vi "Fibre Flow Laser_Control.vi"() -> ()   [LabVIEW 2020]
uses:
  ADAM Client/Sub VIs/ADAM Controls/Update_scan_value.ctl
  Anemometry/Anemometry Sub Vis/File/Setup_Filetype.ctl
  Anemometry/Anemometry Sub Vis/Globals/LDA_global.vi
panel:
  out "BSA IP and Channels":string[](array[string])
  out "Setup String":string
  out "Setup Filename":string
  in  "Update BSA Settings":bool
  out "reference out":refnum<k7>
  in  "SysMon":refnum<k7>(container)
  in  "Stop BSA Monitor":bool
  in  "Start BSA Monitor":bool
  out "Laser Control Error":errorcluster
  out "BSA Error":errorcluster
  in  "Freqency Shift Enable?":bool
  in  "Control Laser":bool
  in  "Mode":T1(ring)
  in  "Set Power (mW)":dbl
  in  "Laser":i32(listbox)
  in  "Seconds before Update":u32=30
  out "Numeric":i32
  in  "stop":bool
  out "Status":string[][](array[string])
  out "Laser Status error":errorcluster
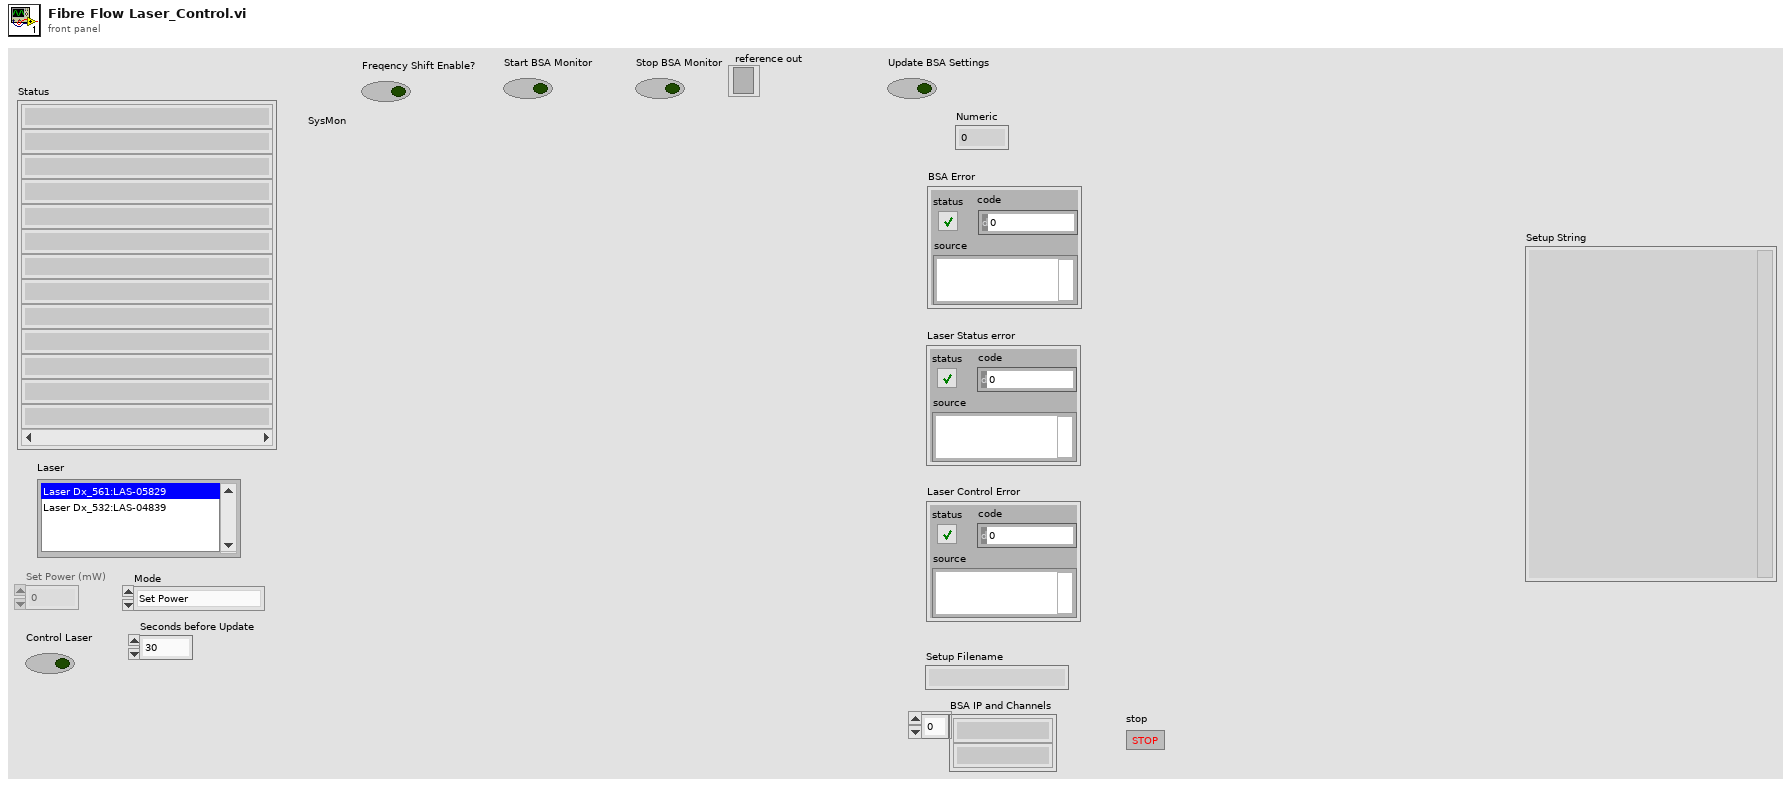
[diagram p1: front panel]
types:
  T1 = enum16{"Set Power", "Turn Laser On", "Turn Laser Off", "Shutter Open", "Shutter Closed", "Attenuated"}
  T2 = typedef "Update_scan_value.ctl" = cluster{"Channel Name":string, "New Value":dbl}
  T3 = enum16{"Zero or one", "One", "Zero or more", "One or more"}
  T4 = typedef "Setup_Filetype.ctl" = enum16{"Measurement Setups", "Calibration Setups", "General", "Results File Plotter Setups", "Speed Calib Tweaks"}
  T5 = enum8{"Enabled", "Disabled", "Disabled and Grayed Out"}
  T6 = typedef "LDA_Channel.ctl" = cluster{"Wavelength (nm)":dbl, "Vel Comp":string, "Max Velocity":dbl, "Min Velocity":dbl, "Max Record length":u16, "Signal gain (dB)":i16, "High voltage":i16, "Optics Conversion Factor":dbl, "Min Record length":u16, "Multiply Velocity by -1":bool, "Signal to Noise Ratio":string, "Validation Ratio":string, "Probe":string, "Laser":string, "BSA":string, "Lense":string, "Beam Separation (mm)":dbl, "Focal Length (mm)":dbl, "COLOUR":u32, "BSA IP":string, "Velocity Range (m/s)":dbl, "Centre Velocity (m/s)":dbl, "Unshifted mW":dbl, "Shifted mW":dbl, "Bandwidth Hz":dbl, "Req Sampling Rate Hz":dbl, "Ch":i32, "CenterFreq Hz":dbl, "Laser IP":string}
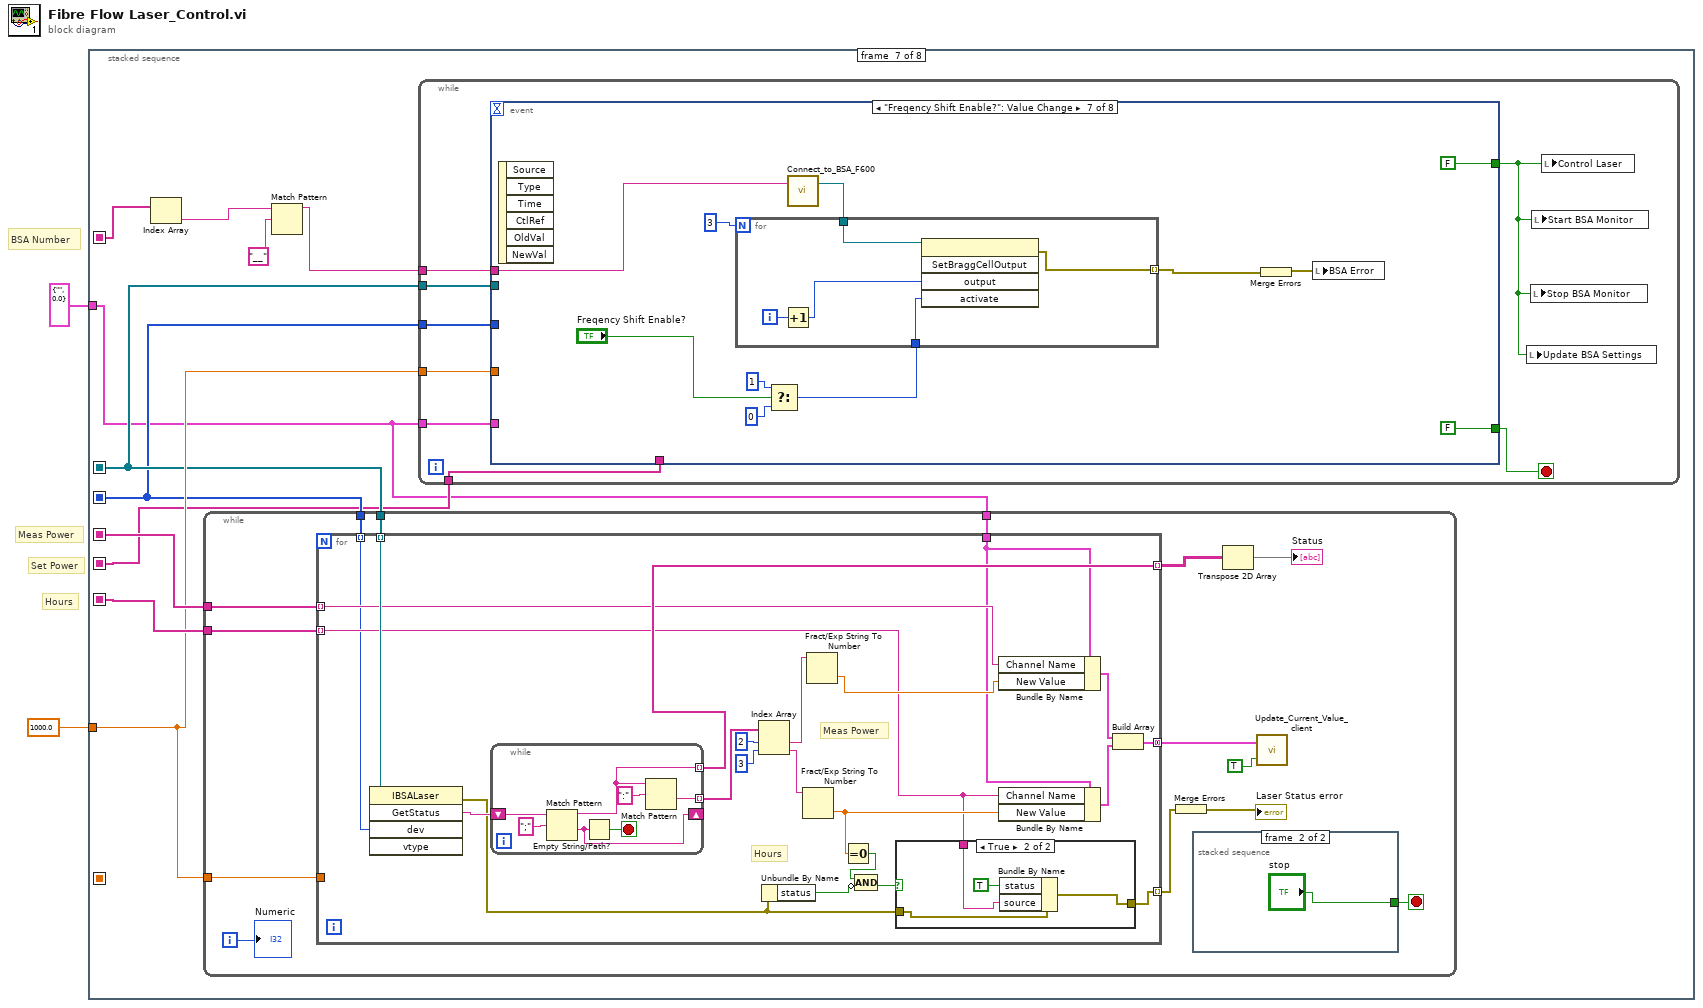
[diagram p0: block diagram]
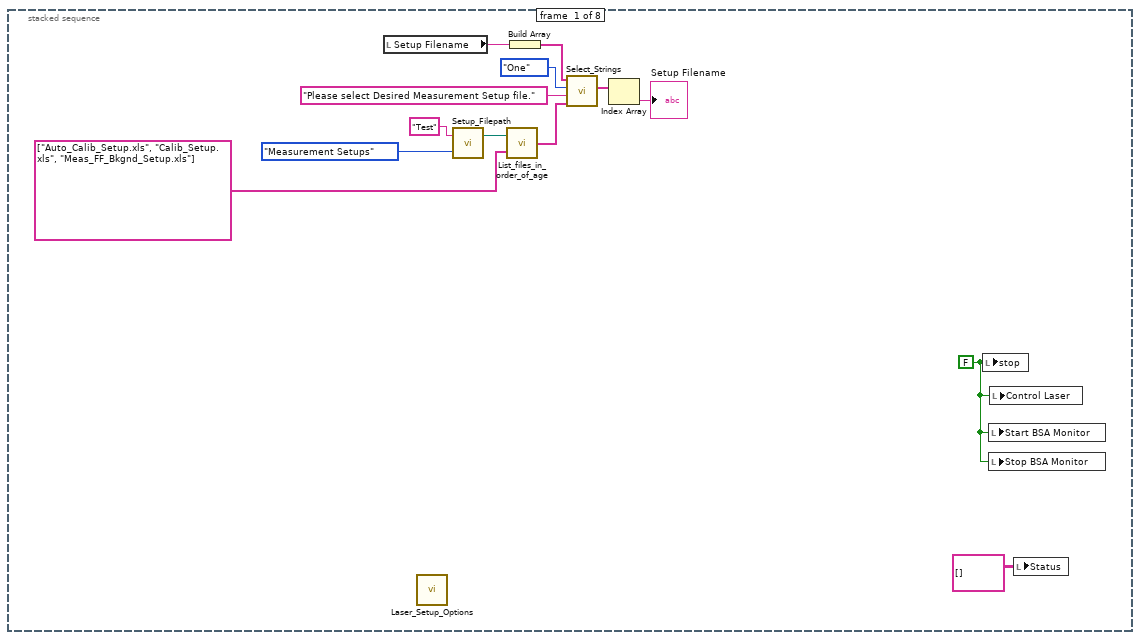
[diagram p2: hidden frame]
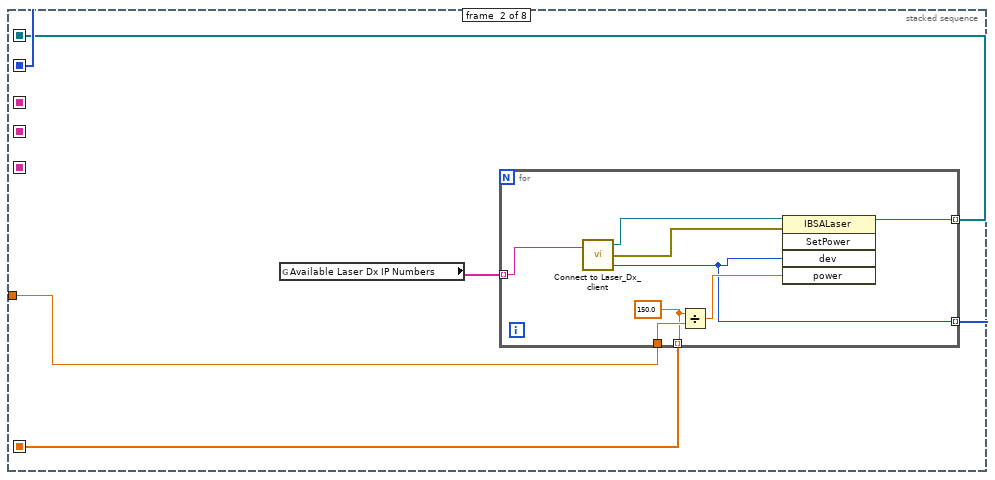
[diagram p3: hidden frame]
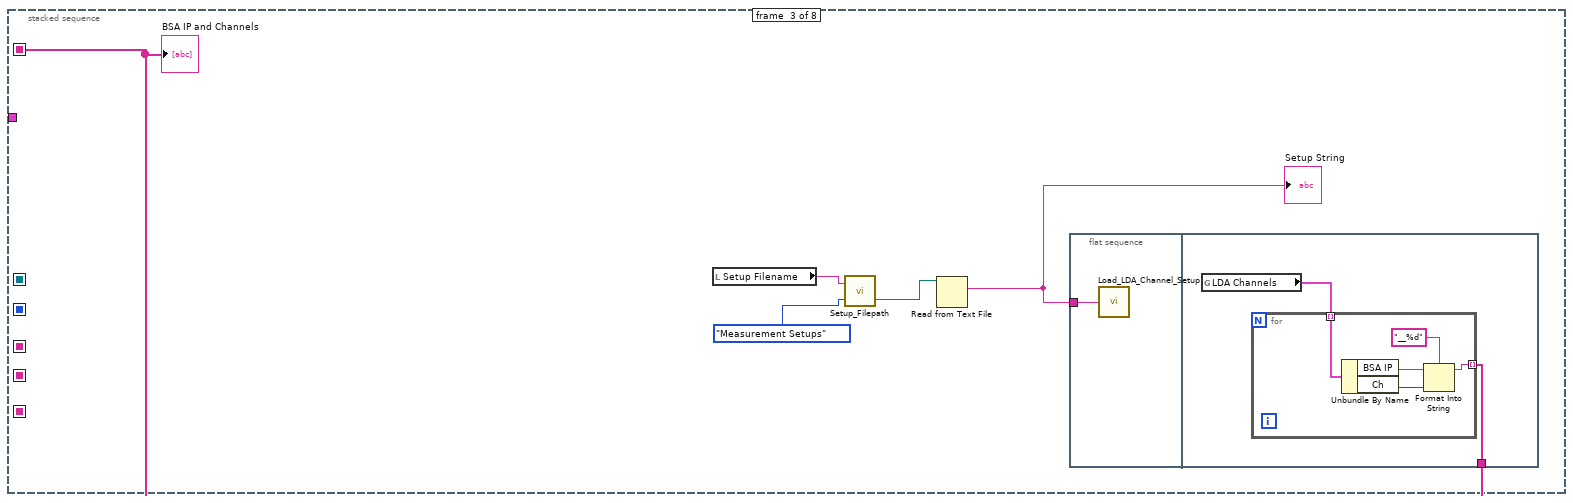
[diagram p4: hidden frame]
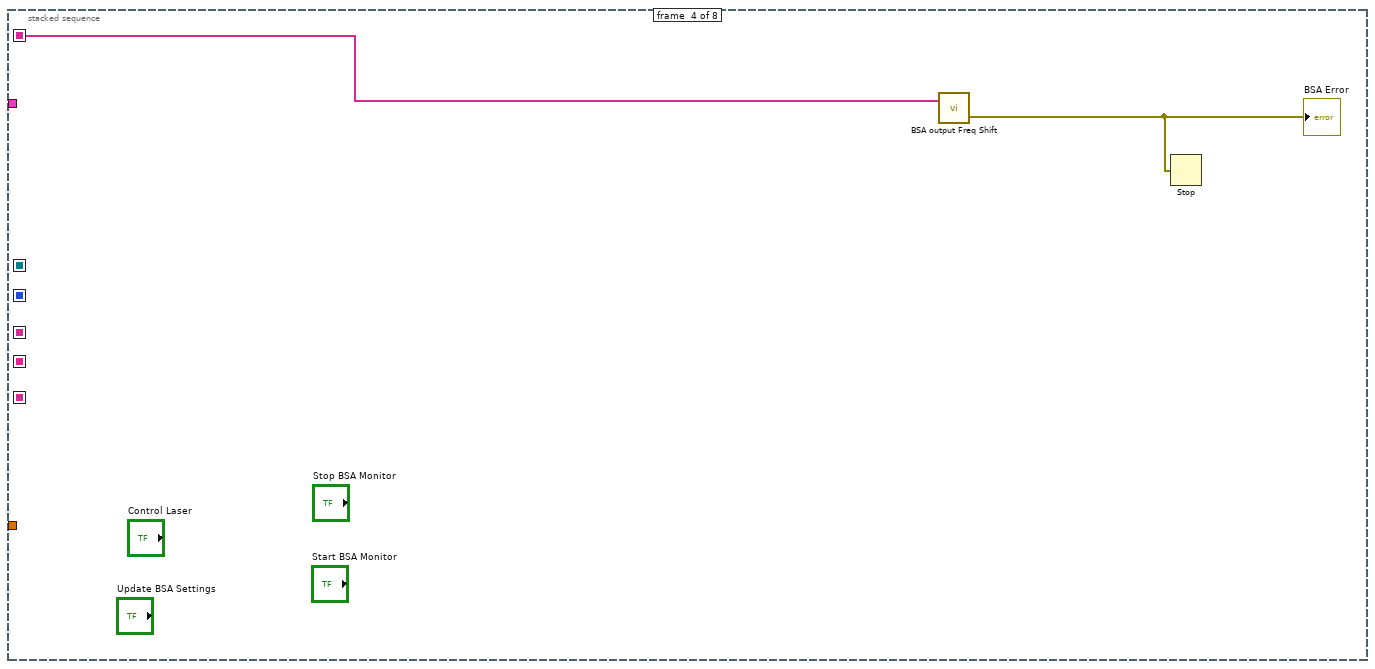
[diagram p5: hidden frame]
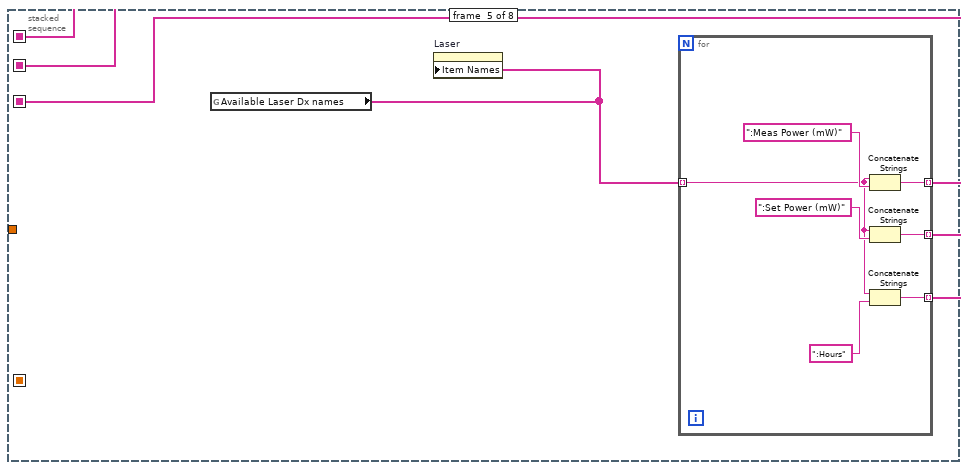
[diagram p6: hidden frame]
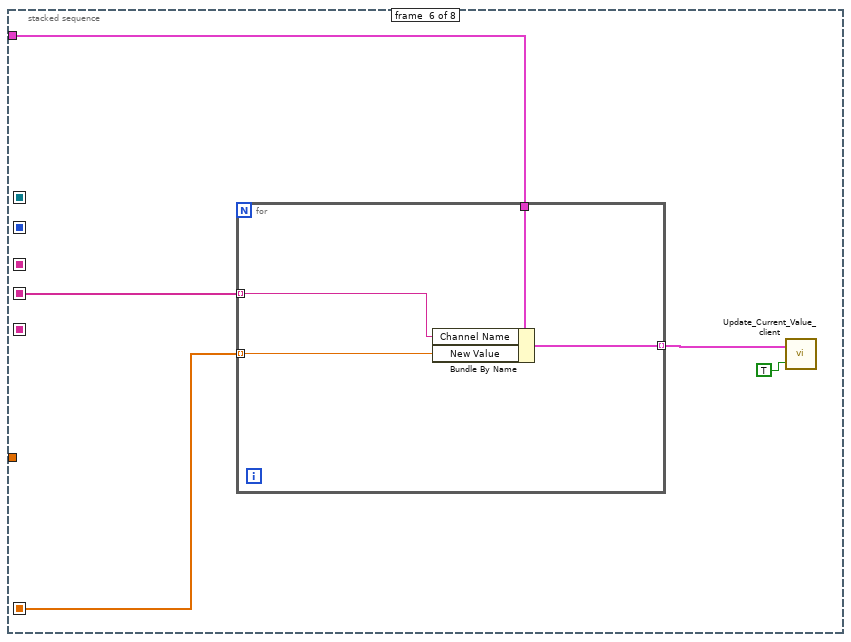
[diagram p7: hidden frame]
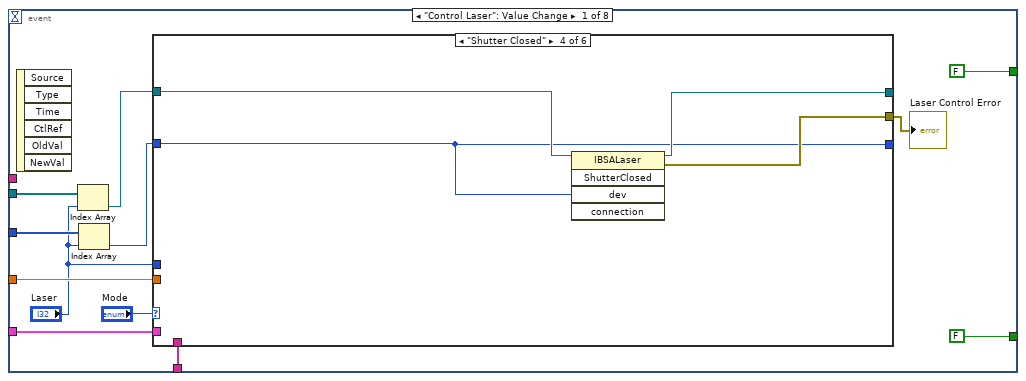
[diagram p8: hidden frame]
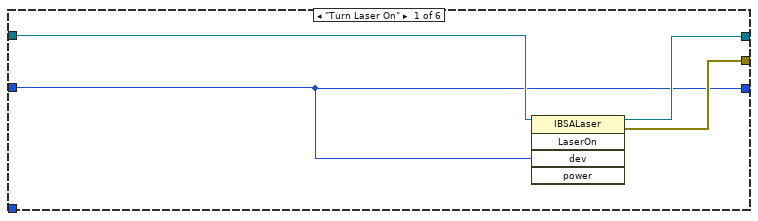
[diagram p9: hidden frame]
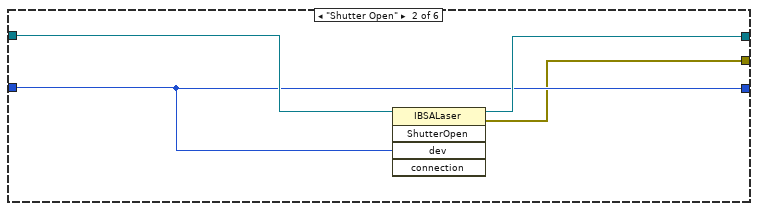
[diagram p10: hidden frame]
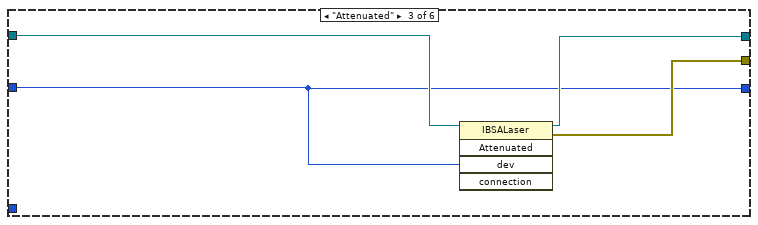
[diagram p11: hidden frame]
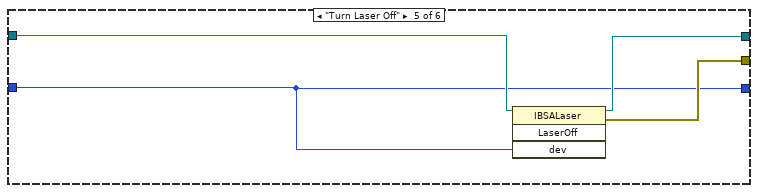
[diagram p12: hidden frame]
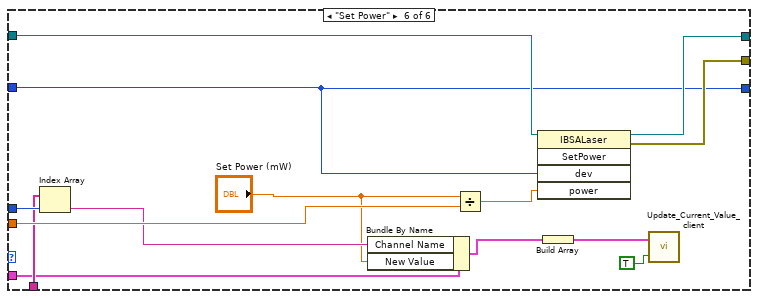
[diagram p13: hidden frame]
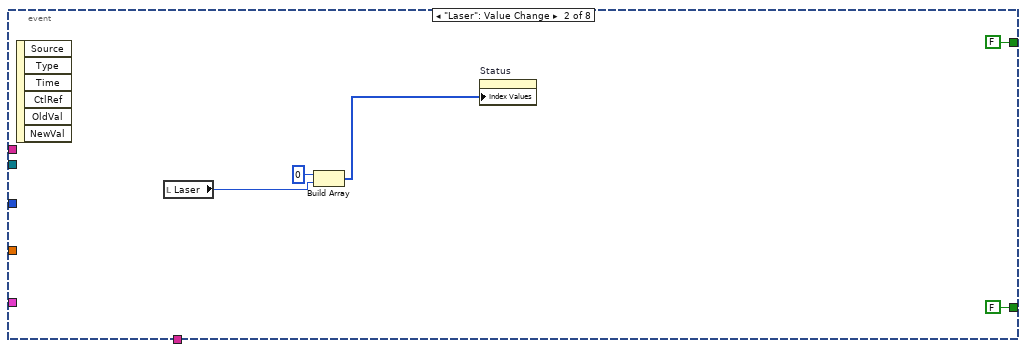
[diagram p14: hidden frame]
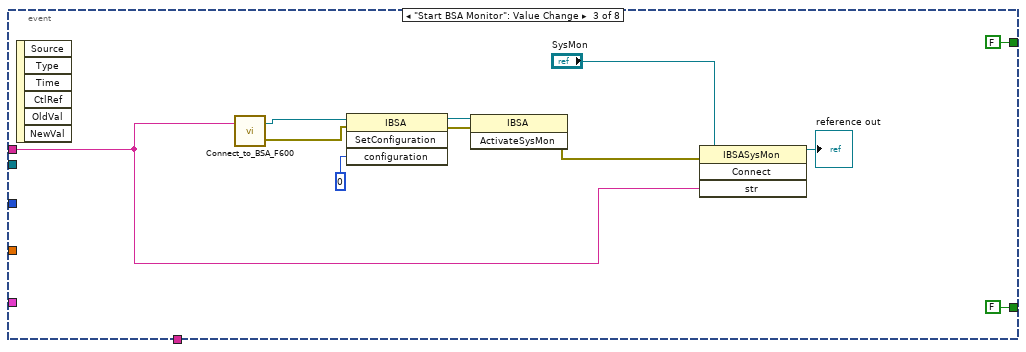
[diagram p15: hidden frame]
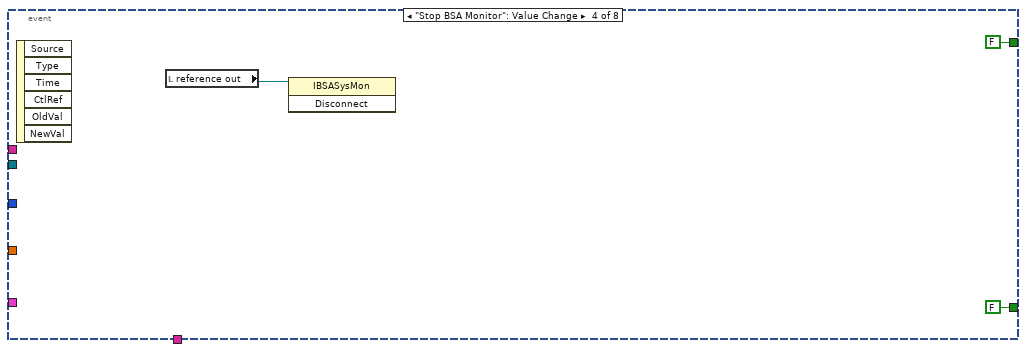
[diagram p16: hidden frame]
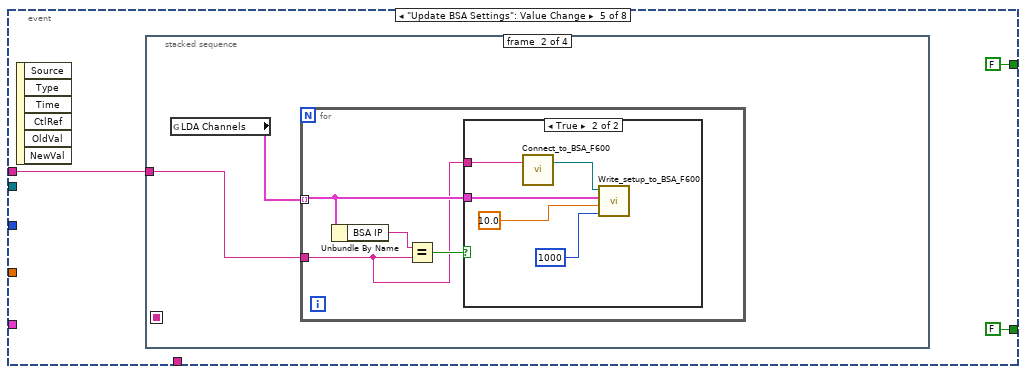
[diagram p17: hidden frame]
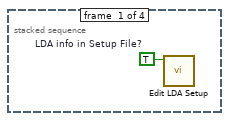
[diagram p18: hidden frame]
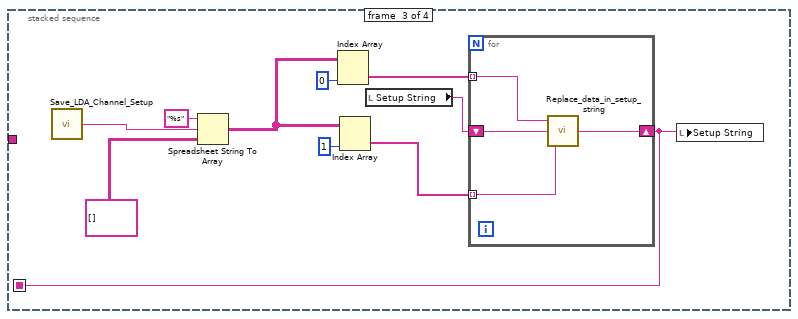
[diagram p20: hidden frame]
diagram:
  # "BSA Number"
  # "Hours"
  # "Set Power"
  # "Meas Power"
  n1 = stacked-sequence {
    seq-local: [_ w16 _ _ _ _ _ _] -> [_ _ _ _ _ _ w71 _]
    seq-local: [_ w20 _ _ _ _ _ _] -> [_ _ _ _ _ _ w70 _]
    seq-local: [_ _ _ _ w47 _ _ _] -> [_ _ _ _ _ _ w74 w268]
    seq-local: [_ _ _ _ w46 _ _ _] -> [_ _ _ _ _ w58 w69 w267]
    seq-local: [_ _ _ _ w45 _ _ _] -> [_ _ _ _ _ _ w73 w266]
    seq-local: [_ w18 _ _ _ _ _ _] -> [_ _ _ _ _ w57 _ _]
    seq-local: [_ _ w30 _ _ _ _ _] -> [_ _ _ w42 _ _ w65 _]
    tunnel: 1000.0 ("y") -> [_ w19 _ _ _ _ w72 _]
    tunnel: T2 {"Channel Name"="", "New Value"=0.0} ("Update Scan Value Cluster") -> [_ _ _ _ _ w55 w68 w264]
    frame #0 {
      w3 = FALSE ("stop")
      n2 = local read "Setup Filename"() -> (w12:string)
      n3 = call "Laser_Setup_Options.vi"() -> ()  [unwired: 5 in, 4 out]
      n4 = call "Setup_Filepath.vi"("Setup File Type"=Setup_Filetype."Measurement Setups", "Filename in"="Test") -> ("Directory"=w15:path)  [unwired: 1 out]
      n5 = call "List_files_in_order_of_age.vi"("Files to Hide"=string[] ["Auto_Calib_Setup.xls", "Calib_Setup.xls", "Meas_FF_Bkgnd_Setup.xls"] ("file names"), "Folder"=w15) -> ("file names"=w14:string[])
      n6 = Build Array(w12) -> (w11:string[])
      n7 = call "Select_Strings.vi"("Available Ch names"=w14, "Message"="Please select Desired Measurement Setup file.", "Selector mode"=T3."One", "Desired Ch names (in)"=w11) -> ("Selected Channel Names"=w13:string[])  [unwired: 2 in, 2 out]
      n8 = Index Array(array=w13) -> (element=→"Setup Filename":string)  [unwired: 1 in]
      n9 = local write "stop"(w3) -> ()
      n10 = local write "Start BSA Monitor"(w3) -> ()
      n11 = local write "Stop BSA Monitor"(w3) -> ()
      n12 = local write "Control Laser"(w3) -> ()
      n13 = local write "Status"(string[][] [] ("Status")) -> ()
    }
    frame #1 {
      n14 = global read "LDA_global.vi" "Available Laser Dx IP Numbers"() -> (w17:string[])
      n15 = for {
        tunnel: w17 -> [w24] mode=indexing
        tunnel: [w28] -> w16 mode=indexing
        tunnel: [w21] -> w20 mode=indexing
        tunnel: w19 -> [w27]
        tunnel: [w25] -> w18 mode=indexing
        w25 = 150.0 ("power")
        n16 = call "Connect to Laser_Dx_client.vi"("Laser IP Number"=w24) -> ("Laser_Dx"=w23:refnum<k7>, "error out"=w22:errorcluster, "Channel"=w21:i64)  [unwired: 1 in]
        n17 = Divide(x=w25, y=w27) -> (x/y=w26:dbl)
        n18 = invoke class="IBSALaser" method="SetPower"(reference=w23, error in=w22, "dev"=w21, "power"=w26) -> (reference out=w28:refnum<k7>)  [unwired: 1 in, 4 out]
      }
    }
    frame #2 {
      n19 = local read "Setup Filename"() -> (w29:string)
      n20 = call "Setup_Filepath.vi"("Setup File Type"=Setup_Filetype."Measurement Setups", "Filename in"=w29) -> ("Filename Out"=w32:path)  [unwired: 1 out]
      n21 = Read from Text File(file (use dialog)=w32) -> (text=w31:string)  [unwired: 3 in, 3 out]
      "Setup String" <- w31
      n22 = flat-sequence {
        tunnel: w31 -> [w34]
        tunnel: [w36] -> w30
        frame #0 {
          n23 = call "Load_LDA_Channel_Setup.vi"("Setup file string"=w34) -> ()  [unwired: 1 in]
        }
        frame #1 {
          n24 = global read "LDA_global.vi" "LDA Channels"() -> (w35:T6[])
          n25 = for {
            tunnel: [w37] -> w36 mode=indexing
            tunnel: w35 -> [w41] mode=indexing
            n26 = Unbundle By Name(w41) -> ("BSA IP"=w39:string, "Ch"=w40:i32)
            n27 = Format Into String(format string="__%d", initial string=w39, w40) -> (resulting string=w37:string)  [unwired: 1 in, 1 out]
          }
        }
      }
      "BSA IP and Channels" <- w30
    }
    frame #3 {
      n28 = call "BSA output Freq Shift.vi"("BSAIP__ChNum"=w42) -> ("BSA Error"=w43:errorcluster)  [unwired: 2 in]
      "BSA Error" <- w43
      n29 = Stop(stop? (T)=w43) -> ()
    }
    frame #4 {
      n30 = global read "LDA_global.vi" "Available Laser Dx names"() -> (w44:string[])
      n31 = property on="Laser" class="LstBox (strict)"("Item Names"=w44) -> ()  [unwired: 2 in, 2 out]
      n32 = for {
        tunnel: [w51] -> w47 mode=indexing
        tunnel: [w50] -> w46 mode=indexing
        tunnel: [w49] -> w45 mode=indexing
        tunnel: w44 -> [w48] mode=indexing
        n33 = Concatenate Strings(w48, ":Meas Power (mW)" ("string")) -> (w51:string)
        n34 = Concatenate Strings(w48, ":Set Power (mW)" ("string")) -> (w50:string)
        n35 = Concatenate Strings(w48, ":Hours" ("string")) -> (w49:string)
      }
    }
    frame #5 {
      n36 = for {
        tunnel: w58 -> [w63] mode=indexing
        tunnel: w57 -> [w62] mode=indexing
        tunnel: [w61] -> w56 mode=indexing
        tunnel: w55 -> [w60]
        n37 = Bundle By Name(cluster=w60, "Channel Name"=w63, "New Value"=w62) -> (w61:T2)
      }
      n38 = call "Update_Current_Value_client.vi"("Don't Bother with check?"=TRUE, "Update array in"=w56) -> ()
    }
    frame #6 {
      n39 = Index Array(array=w65) -> (element=w66:string)  [unwired: 1 in]
      n40 = while {
        tunnel: w71 -> [w222]
        tunnel: w70 -> [w221]
        tunnel: w72 -> [w220]
        tunnel: w74 -> [w217]
        tunnel: w73 -> [w216]
        tunnel: w68 -> [w214]
        i -> [w218]
        stop <- w215 stop-if-true
        n41 = for {
          tunnel: [w249] -> w224 mode=concatenating
          tunnel: w222 -> [w239] mode=indexing
          tunnel: w221 -> [w229] mode=indexing
          tunnel: w220 -> [_]
          tunnel: [w240] -> w219 mode=indexing
          tunnel: w217 -> [w238] mode=indexing
          tunnel: w216 -> [w234] mode=indexing
          tunnel: w214 -> [w237]
          tunnel: [w235] -> w213 mode=indexing
          # "Meas Power"
          # "Hours"
          n42 = invoke class="IBSALaser" method="GetStatus"(reference=w239, "dev"=w229) -> (error out=w233:errorcluster, "GetStatus"=w241:string)  [unwired: 3 in, 3 out]
          n43 = while {
            shift-right: [w259] -> _
            shift-left: w241 -> [w261]
            tunnel: [w258] -> w240 mode=indexing
            tunnel: [w256] -> w242 mode=indexing
            stop <- w260 stop-if-true
            n44 = Match Pattern(string=w261, regular expression=";") -> (before substring=w258:string, after substring=w259:string)  [unwired: 1 in, 2 out]
            n45 = Empty String/Path?(string/path=w259) -> (empty?=w260:bool)
            n46 = Match Pattern(string=w258, regular expression=":") -> (after substring=w256:string)  [unwired: 1 in, 3 out]
          }
          n47 = Index Array(array=w242, index #1=2 ("index"), index #2=3 ("index")) -> (element #1=w245:string, element #2=w247:string)
          n48 = Unbundle By Name(w233) -> ("status"=w232:bool)
          n49 = Fract/Exp String To Number(string=w247) -> (number=w236:dbl)  [unwired: 3 in, 1 out]
          n50 = Fract/Exp String To Number(string=w245) -> (number=w246:dbl)  [unwired: 3 in, 1 out]
          n51 = Equal To 0?(x=w236) -> (x = 0?=w231:bool)
          n52 = Compound Arithmetic op=AND(w231, invert w232) -> (w230:bool)
          n53 = case shown="True" w230 {
            tunnel: [w251 w252] -> w235
            tunnel: w233 -> [w251 w255]
            tunnel: w234 -> [_ w253]
            frame False {
            }
            frame True {
              n54 = Bundle By Name(cluster=w255, "status"=TRUE, "source"=w253) -> (w252:errorcluster)
            }
          }
          n55 = Bundle By Name(cluster=w237, "Channel Name"=w238, "New Value"=w246) -> (w248:T2)
          n56 = Bundle By Name(cluster=w237, "Channel Name"=w234, "New Value"=w236) -> (w250:T2)
          n57 = Build Array(w248, w250) -> (w249:T2[])
        }
        n58 = Merge Errors(w213) -> (→"Laser Status error":errorcluster)
        n59 = stacked-sequence {
          tunnel: [_ "stop"] -> w215
          frame #0 {
            n60 = Multiply(x="Seconds before Update", y=u32 1000 ("millisecond timer value")) -> (x*y=w227:u32)
            n61 = Wait Until Next ms Multiple(millisecond multiple=w227) -> ()  [unwired: 1 out]
          }
          frame #1 {
          }
        }
        n62 = Transpose 2D Array(2D array=w219) -> (transposed array=→"Status":string[][])
        n63 = call "Update_Current_Value_client.vi"("Don't Bother with check?"=TRUE, "Update array in"=w224) -> ()
        "Numeric" <- w218
      }
      n64 = Match Pattern(string=w66, regular expression="__" ("string")) -> (before substring=w64:string)  [unwired: 1 in, 3 out]
      n65 = while {
        tunnel: w72 -> [w82]
        tunnel: w71 -> [w81]
        tunnel: w70 -> [w80]
        tunnel: w69 -> [w79]
        tunnel: w68 -> [w78]
        tunnel: w64 -> [w77]
        stop <- w76 stop-if-true
        n66 = event shown="[6] \"Freqency Shift Enable?\": Value Change" {
          selector: _ -> [_ _ _ _ _ _ _ _]
          dyn-events: _ -> [_ _ _ _ _ _ _ _]
          timeout: _ -> [_ _ _ _ _ _ _ _]
          tunnel: w82 -> [w94 _ _ _ _ _ _ _]
          tunnel: w81 -> [w92 _ _ _ _ _ _ _]
          tunnel: w80 -> [w91 _ _ _ _ _ _ _]
          tunnel: [FALSE FALSE FALSE FALSE FALSE FALSE FALSE TRUE] -> w76
          tunnel: w79 -> [w86 _ _ _ _ _ _ _]
          tunnel: w78 -> [w85 _ _ _ _ _ _ _]
          tunnel: [FALSE ("Control Laser") FALSE ("Control Laser") FALSE ("Control Laser") FALSE ("Control Laser") FALSE ("Control Laser") FALSE ("Control Laser") FALSE ("Control Laser") FALSE ("Control Laser")] -> w75
          tunnel: w77 -> [_ _ w136 _ w150 _ w194 _]
          event "Control Laser": Value Change {
            n67 = event-data() -> ()  [unwired: 1 in, 6 out]
            n68 = Index Array(array=w92, index="Laser") -> (element=w90:refnum<k7>)
            n69 = Index Array(array=w91, index="Laser") -> (element=w89:i64)
            n70 = case shown="\"Shutter Closed\"" "Mode" {
              tunnel: [w97 w101 w105 w109 w113 w127] -> _
              tunnel: [w96 w99 w104 w108 w112 w126] -> w84
              tunnel: [w95 w100 w103 w107 w111 w125] -> _
              tunnel: w90 -> [w98 w102 w106 w110 w114 w128]
              tunnel: w89 -> [w95 w100 w103 w107 w111 w125]
              tunnel: w94 -> [_ _ _ _ _ w124]
              tunnel: "Laser" -> [_ _ _ _ _ w122]
              tunnel: w86 -> [_ _ _ _ _ w121]
              tunnel: w85 -> [_ _ _ _ _ w117]
              frame "Turn Laser On" {
                n71 = invoke class="IBSALaser" method="LaserOn"(reference=w98, "dev"=w95) -> (reference out=w97:refnum<k7>, error out=w96:errorcluster)  [unwired: 3 in, 3 out]
              }
              frame "Shutter Open" {
                n72 = invoke class="IBSALaser" method="ShutterOpen"(reference=w102, "dev"=w100) -> (reference out=w101:refnum<k7>, error out=w99:errorcluster)  [unwired: 3 in, 3 out]
              }
              frame "Attenuated" {
                n73 = invoke class="IBSALaser" method="Attenuated"(reference=w106, "dev"=w103) -> (reference out=w105:refnum<k7>, error out=w104:errorcluster)  [unwired: 3 in, 3 out]
              }
              frame "Shutter Closed" {
                n74 = invoke class="IBSALaser" method="ShutterClosed"(reference=w110, "dev"=w107) -> (reference out=w109:refnum<k7>, error out=w108:errorcluster)  [unwired: 3 in, 3 out]
              }
              frame "Turn Laser Off" {
                n75 = invoke class="IBSALaser" method="LaserOff"(reference=w114, "dev"=w111) -> (reference out=w113:refnum<k7>, error out=w112:errorcluster)  [unwired: 2 in, 2 out]
              }
              frame "Set Power" {
                n76 = Index Array(array=w121, index=w122) -> (element=w119:string)
                n77 = Bundle By Name(cluster=w117, "Channel Name"=w119, "New Value"="Set Power (mW)") -> (w116:T2)
                n78 = Divide(x="Set Power (mW)", y=w124) -> (x/y=w123:dbl)
                n79 = invoke class="IBSALaser" method="SetPower"(reference=w128, "dev"=w125, "power"=w123) -> (reference out=w127:refnum<k7>, error out=w126:errorcluster)  [unwired: 2 in, 3 out]
                n80 = Build Array(w116) -> (w115:T2[])
                n81 = call "Update_Current_Value_client.vi"("Don't Bother with check?"=TRUE, "Update array in"=w115) -> ()
              }
            }
            "Laser Control Error" <- w84
          }
          event "Laser": Value Change {
            n82 = event-data() -> ()  [unwired: 1 in, 6 out]
            n83 = local read "Laser"() -> (w131:i32)
            n84 = Build Array(0 ("element"), w131) -> (w130:i32[])
            n85 = property on="Status" class="Arr (strict)"("Index Values"=w130) -> ()  [unwired: 2 in, 2 out]
          }
          event "Start BSA Monitor": Value Change {
            n86 = event-data() -> ()  [unwired: 1 in, 6 out]
            n87 = call "Connect_to_BSA_F600.vi"("BSA IP Number"=w136) -> ("error out"=w134:errorcluster, "F600"=w135:refnum<k7>)  [unwired: 1 in]
            n88 = invoke class="IBSA" method="SetConfiguration"(reference=w135, error in=w134, "configuration"=0 ("config")) -> (reference out=w142:refnum<k7>, error out=w144:errorcluster)  [unwired: 1 in, 2 out]
            n89 = invoke class="IBSA" method="ActivateSysMon"(reference=w142, error in=w144) -> (error out=w141:errorcluster)  [unwired: 1 in, 2 out]
            n90 = invoke class="IBSASysMon" method="Connect"(reference="SysMon", error in=w141, "str"=w136) -> (reference out=→"reference out":refnum<k7>)  [unwired: 1 in, 3 out]
          }
          event "Stop BSA Monitor": Value Change {
            n91 = event-data() -> ()  [unwired: 1 in, 6 out]
            n92 = local read "reference out"() -> (w147:refnum<k7>)
            n93 = invoke class="IBSASysMon" method="Disconnect"(reference=w147) -> ()  [unwired: 2 in, 3 out]
          }
          event "Update BSA Settings": Value Change {
            n94 = event-data() -> ()  [unwired: 1 in, 6 out]
            n95 = stacked-sequence {
              seq-local: [_ _ w163 _] -> [_ _ _ w177]
              tunnel: w150 -> [_ w152 _ _]
              frame #0 {
                w151 = TRUE  # LDA info in Setup File?
                n96 = call "Edit LDA Setup.vi"("LDA info in Setup File?"=w151) -> ()  [unwired: 11 in]
              }
              frame #1 {
                n97 = global read "LDA_global.vi" "LDA Channels"() -> (w153:T6[])
                n98 = for {
                  tunnel: w153 -> [w157] mode=indexing
                  tunnel: w152 -> [w154]
                  n99 = Unbundle By Name(w157) -> ("BSA IP"=w156:string)
                  n100 = Equal?(x=w156, y=w154) -> (x = y?=w155:bool)
                  n101 = case shown="True" w155 {
                    tunnel: w157 -> [_ w160]
                    tunnel: w154 -> [_ w159]
                    frame False {
                    }
                    frame True {
                      n102 = call "Connect_to_BSA_F600.vi"("BSA IP Number"=w159) -> ("F600"=w158:refnum<k7>)  [unwired: 1 in, 1 out]
                      n103 = call "Write_setup_to_BSA_F600.vi"("No Of Samples"=1000, "Time (s)"=sgl 10.0, "BSA Setup In"=w160, "BSACtrl.IBSA F600"=w158) -> ()  [unwired: 3 out]
                    }
                  }
                }
              }
              frame #2 {
                n104 = call "Save_LDA_Channel_Setup.vi"() -> ("Setup file string"=w172:string)  [unwired: 1 in]
                n105 = Spreadsheet String To Array(format string="%s", spreadsheet string=w172, array type (2D Dbl)=string[][] []) -> (array=w171:string[][])  [unwired: 1 in]
                n106 = Index Array(array=w171, index (col)=0 ("disabled index (col)")) -> (element=w170:string[])  [unwired: 1 in]
                n107 = Index Array(array=w171, index (col)=1 ("disabled index (col)")) -> (element=w169:string[])  [unwired: 1 in]
                n108 = local read "Setup String"() -> (w168:string)
                n109 = for {
                  tunnel: w170 -> [w176] mode=indexing
                  tunnel: w169 -> [w174] mode=indexing
                  shift-right: [w173] -> w163
                  shift-left: w168 -> [w175]
                  n110 = call "Replace_data_in_setup_string.vi"("New data string"=w174, "Input string"=w175, "Variable name"=w176) -> ("Appended string"=w173:string)
                }
                n111 = local write "Setup String"(w163) -> ()
              }
              frame #3 {
                w179 = "Current_Setup.xls"
                w178 = Setup_Filetype."Measurement Setups" ("Setup File Type")
                n112 = local read "Setup Filename"() -> (w181:string)
                n113 = Not Equal?(x=w179, y=w181) -> (x != y?=w180:bool)
                n114 = call "Setup_Filepath.vi"("Setup File Type"=w178, "Filename in"=w181) -> ("Filename Out"=w182:path)  [unwired: 1 out]
                n115 = Write to Text File(file (use dialog)=w182, text=w177) -> ()  [unwired: 2 in, 3 out]
                n116 = case shown="True" w180 {
                  tunnel: w179 -> [_ w186]
                  tunnel: w178 -> [_ w185]
                  tunnel: w177 -> [_ w184]
                  frame False {
                  }
                  frame True {
                    n117 = call "Setup_Filepath.vi"("Setup File Type"=w185, "Filename in"=w186) -> ("Filename Out"=w183:path)  [unwired: 1 out]
                    n118 = Write to Text File(file (use dialog)=w183, text=w184) -> ()  [unwired: 2 in, 3 out]
                  }
                }
              }
            }
          }
          event "Mode": Value Change {
            n119 = event-data() -> ()  [unwired: 1 in, 6 out]
            n120 = local read "Mode"() -> (w190:T1)
            n121 = case shown="Default" w190 {
              tunnel: [T5."Enabled" ("Disabled") T5."Disabled and Grayed Out" ("Disabled")] -> w189
              frame "Set Power" {
              }
              frame Default {
              }
            }
            n122 = property on="Set Power (mW)" class="DigNum (strict)"("DisabledEnum"=w189) -> ()  [unwired: 2 in, 2 out]
          }
          event "Freqency Shift Enable?": Value Change {
            n123 = event-data() -> ()  [unwired: 1 in, 6 out]
            n124 = Select(t=1 ("activate"), s="Freqency Shift Enable?", f=0) -> (s? t:f=w200:i32)
            n125 = call "Connect_to_BSA_F600.vi"("BSA IP Number"=w194) -> ("F600"=w193:refnum<k7>)  [unwired: 1 in, 1 out]
            n126 = for {
              N: 3 -> [_]
              tunnel: w200 -> [w206]
              tunnel: w193 -> [w205]
              tunnel: [w204] -> w196 mode=indexing
              i -> [w207]
              n127 = Increment(x=w207) -> (x+1=w208:i32)
              n128 = invoke method="SetBraggCellOutput"(reference=w205, "output"=w208, "activate"=w206) -> (error out=w204:errorcluster)  [unwired: 2 in, 4 out]
            }
            n129 = Merge Errors(w196) -> (w195:errorcluster)
            n130 = local write "BSA Error"(w195) -> ()
          }
          event "stop": Value Change {
            n131 = event-data() -> ()  [unwired: 1 in, 6 out]
          }
        }
        n132 = local write "Update BSA Settings"(w75) -> ()
        n133 = local write "Stop BSA Monitor"(w75) -> ()
        n134 = local write "Start BSA Monitor"(w75) -> ()
        n135 = local write "Control Laser"(w75) -> ()
      }
    }
    frame #7 {
      n136 = Build Array (concatenate)(w268, w267, w266) -> (w265:string[])
      n137 = for {
        tunnel: w265 -> [w273] mode=indexing
        tunnel: w264 -> [w271]
        tunnel: [w270] -> w263 mode=indexing
        n138 = Bundle By Name(cluster=w271, "Channel Name"=w273, "New Value"=nan) -> (w270:T2)
      }
      n139 = call "Update_Current_Value_client.vi"("Don't Bother with check?"=TRUE, "Update array in"=w263) -> ()
    }
  }
